vi "Myrio_9.vi"() -> ()   [LabVIEW 2012]
uses:
  SubVIs/LVPresent_Globals.vi
panel:
  in  "Solution 2":bool
  # "Program an LED to Blink"
  # "Now modify the code you have already written to make the LED blink 5 times.\n\nYou may need to use the \"Wait\" function and a for loop in order to do this."
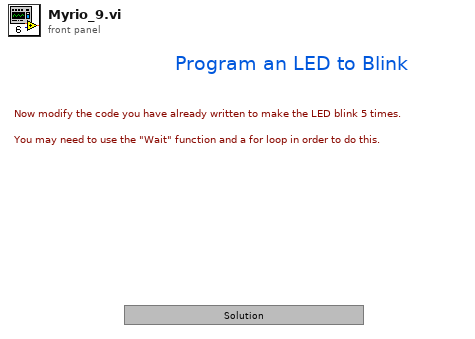
[diagram p1: front panel]
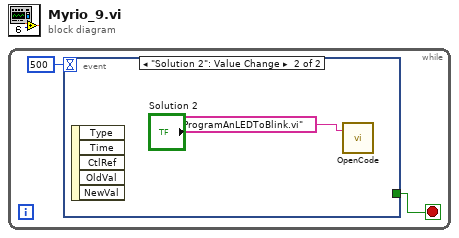
[diagram p0: block diagram]
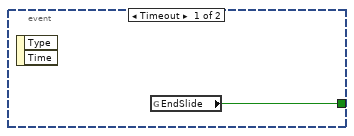
[diagram p2: hidden frame]
diagram:
  n1 = while {
    stop <- w2 stop-if-true
    n2 = event shown="[1] \"Solution 2\": Value Change" {
      selector: _ -> [_ _]
      dyn-events: _ -> [_ _]
      timeout: 500 -> [_ _]
      tunnel: [w3 _] -> w2
      event Timeout {
        n3 = event-data() -> ()  [unwired: 1 in, 2 out]
        n4 = global read "LVPresent_Globals.vi" "EndSlide"() -> (w3:bool)
      }
      event "Solution 2": Value Change {
        n5 = event-data() -> ()  [unwired: 1 in, 5 out]
        n6 = call <userlib>:"OpenCode.vi"("Code name"="ProgramAnLEDToBlink.vi") -> ()  [unwired: 3 in]
      }
    }
  }
